vi "Read Attributes.vi"(11 "Caller Notice Msg":refnum<class "Caller Notice Msg.lvclass">) -> (2 "Payload":T1)   [LabVIEW 2020, in "Generic Actor.lvlib" / "Caller Notice Msg.lvclass"]
uses:
  Caller Notice Msg.lvclass
  Caller Notice Msg.lvclass/Caller Notice Msg.ctl
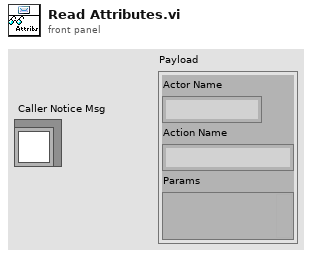
[diagram p1: front panel]
types:
  T1 = cluster{"Actor Name":string, "Action Name":string, "Params":variant}
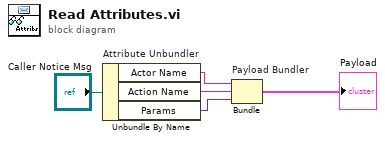
[diagram p0: block diagram]
diagram:
  n1 = Unbundle By Name "Attribute Unbundler"("Caller Notice Msg") -> ("Actor Name"=w3:string, "Action Name"=w2:string, "Params"=w1:variant)
  n2 = Bundle "Payload Bundler"("Actor Name"=w3, "Action Name"=w2, "Params"=w1) -> (→"Payload":T1)  [unwired: 1 in]
